vi "Read Data Source.vi"(8 "error in (no error)":errorcluster, 11 "Data Source Name":string) -> (0 "error out":errorcluster, 3 "Connection Information":T1)   [LabVIEW 2020]
uses:
  ctl/Connection Information.ctl
  <vilib>/Utility/config.llb/Read Key (String).vi
  <vilib>/Utility/config.llb/Read Key (Double).vi
  <vilib>/Utility/config.llb/Read Key (Boolean).vi
  <vilib>/Utility/config.llb/Read Key (Path).vi
  <vilib>/Utility/config.llb/NI_LVConfig.lvlib
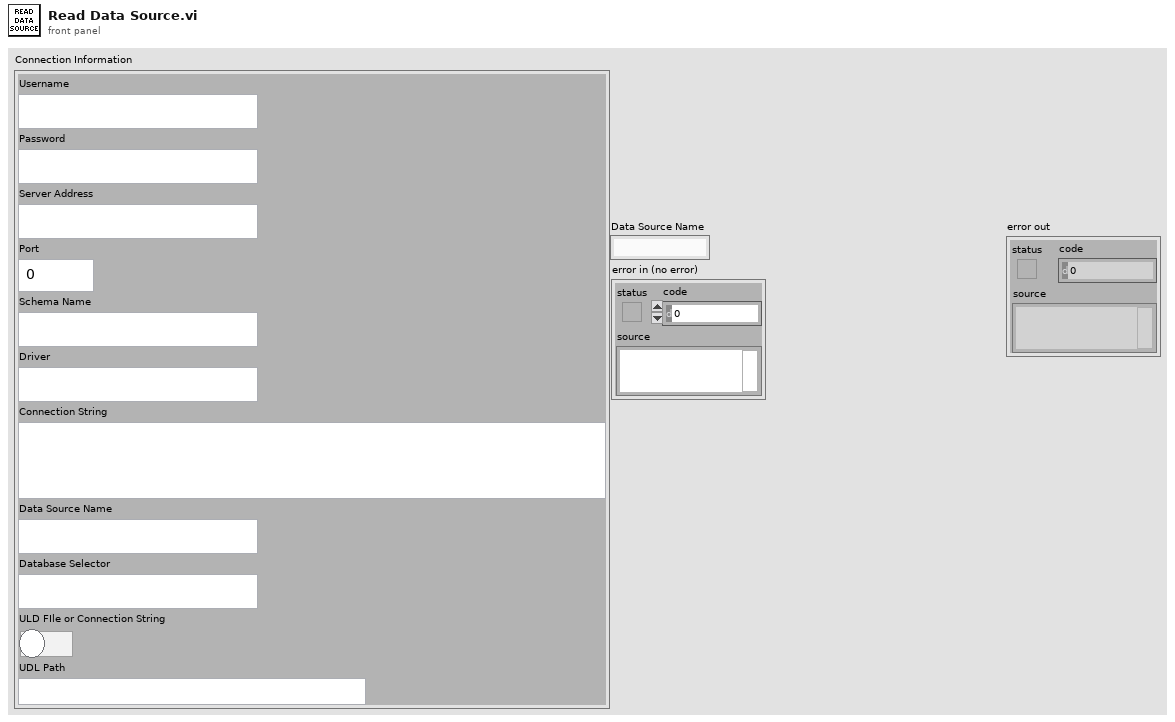
[diagram p1: front panel]
types:
  T1 = typedef "Connection Information.ctl" = cluster{"Username":string, "Password":string, "Server Address":string, "Port":u32, "Schema Name":string, "Driver":string, "Connection String":string, "Data Source Name":string, "Database Selector":string, "ULD FIle or Connection String":bool, "UDL Path":path}
  T2 = typedef "NI_LVConfig.lvlib/Config Data RefNum.ctl" = refnum<k1>
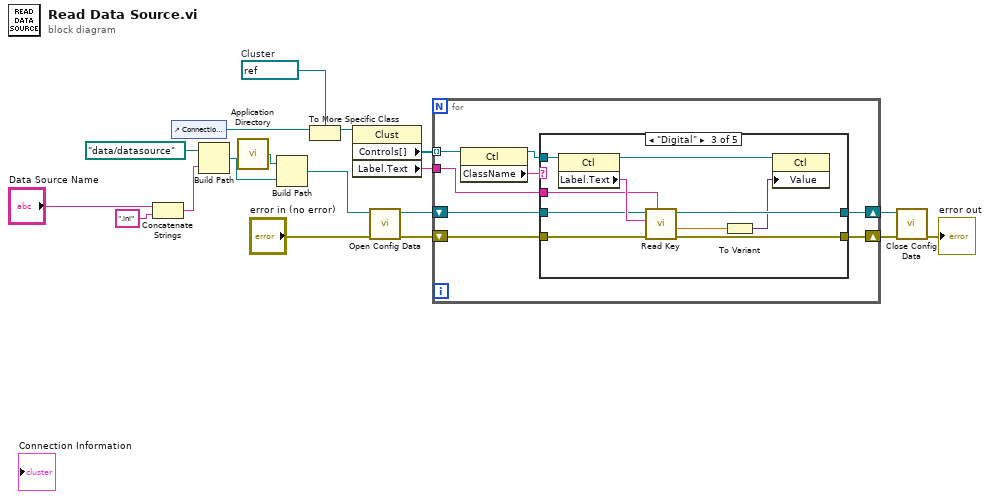
[diagram p0: block diagram]
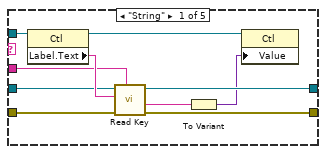
[diagram p2: hidden frame]
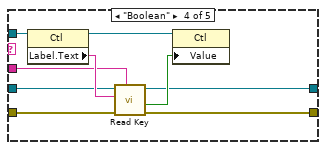
[diagram p4: hidden frame]
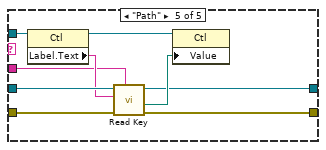
[diagram p5: hidden frame]
diagram:
  w5 = refnum<vi> refnum  # Cluster
  n1 = Concatenate Strings("Data Source Name", ".ini" ("string")) -> (w8:string)
  n2 = control-ref of="Connection Information"() -> (w1:refnum<vi>)
  n3 = Build Path(base path=path "data/datasource", name or relative path=w8) -> (appended path=w10:path)
  n4 = call <vilib>:"Application Directory.vi"() -> ("Application Directory"=w18:path)
  n5 = Build Path(base path=w18, name or relative path=w10) -> (appended path=w17:path)
  n6 = To More Specific Class(target class=w5, reference=w1) -> (specific class reference=w4:refnum<vi>)  [unwired: 1 in, 1 out]
  n7 = property class="Clust"(reference=w4) -> ("Controls[]"=w3:refnum<vi>[], "Label.Text"=w2:string)  [unwired: 1 in, 2 out]
  n8 = call <vilib>:"Open Config Data.vi"("error in (no error)"="error in (no error)", "configuration file path"=w17) -> ("error out"=w13:errorcluster, "refnum"=w14:T2)  [unwired: 7 in, 1 out]
  n9 = for {
    tunnel: w3 -> [w20] mode=indexing
    tunnel: w2 -> [w19]
    shift-right: [w22] -> w15
    shift-left: w14 -> [w25]
    shift-right: [w21] -> w16
    shift-left: w13 -> [w24]
    n10 = property class="Ctl"(reference=w20) -> (reference out=w23:refnum<vi>, "ClassName"=w26:string)  [unwired: 1 in, 1 out]
    n11 = case shown="\"Digital\"" w26 {
      tunnel: w25 -> [w32 w38 w45 w53 w65]
      tunnel: w24 -> [w33 w37 w44 w52 w64]
      tunnel: w23 -> [w34 _ w46 w54 w66]
      tunnel: [w31 w38 w43 w51 w60] -> w22
      tunnel: [w30 w37 w42 w50 w59] -> w21
      tunnel: w19 -> [w27 _ w41 w49 w58]
      frame "String" {
        n12 = property class="Ctl"(reference=w34) -> (reference out=w35:refnum<vi>, "Label.Text"=w36:string)  [unwired: 1 in, 1 out]
        n13 = call-poly <vilib>:"Read Key.vi"("section"=w27, "error in (no error)"=w33, "key"=w36, "refnum"=w32) -> ("error out"=w30:errorcluster, "value"=w28:string, "refnum out"=w31:T2)  [unwired: 4 in, 1 out]
        n14 = To Variant(anything=w28) -> (Variant=w29:variant)
        n15 = property class="Ctl"(reference=w35, "Value"=w29) -> ()  [unwired: 1 in, 2 out]
      }
      frame "", Default {
      }
      frame "Digital" {
        n16 = property class="Ctl"(reference=w46) -> (reference out=w47:refnum<vi>, "Label.Text"=w48:string)  [unwired: 1 in, 1 out]
        n17 = call-poly <vilib>:"Read Key.vi"("section"=w41, "error in (no error)"=w44, "key"=w48, "refnum"=w45) -> ("error out"=w42:errorcluster, "value"=w39:dbl, "refnum out"=w43:T2)  [unwired: 4 in, 1 out]
        n18 = To Variant(anything=w39) -> (Variant=w40:variant)
        n19 = property class="Ctl"(reference=w47, "Value"=w40) -> ()  [unwired: 1 in, 2 out]
      }
      frame "Boolean" {
        n20 = property class="Ctl"(reference=w54) -> (reference out=w56:refnum<vi>, "Label.Text"=w57:string)  [unwired: 1 in, 1 out]
        n21 = call-poly <vilib>:"Read Key.vi"("section"=w49, "error in (no error)"=w52, "key"=w57, "refnum"=w53) -> ("error out"=w50:errorcluster, "value"=w55:bool, "refnum out"=w51:T2)  [unwired: 4 in, 1 out]
        n22 = property class="Ctl"(reference=w56, "Value"=w55) -> ()  [unwired: 1 in, 2 out]
      }
      frame "Path" {
        n23 = property class="Ctl"(reference=w66) -> (reference out=w62:refnum<vi>, "Label.Text"=w63:string)  [unwired: 1 in, 1 out]
        n24 = call-poly <vilib>:"Read Key.vi"("section"=w58, "error in (no error)"=w64, "key"=w63, "refnum"=w65) -> ("error out"=w59:errorcluster, "value"=w61:path, "refnum out"=w60:T2)  [unwired: 4 in, 1 out]
        n25 = property class="Ctl"(reference=w62, "Value"=w61) -> ()  [unwired: 1 in, 2 out]
      }
    }
  }
  n26 = call <vilib>:"Close Config Data.vi"("error in (no error)"=w16, "refnum"=w15) -> ("error out"=→"error out":errorcluster)  [unwired: 8 in, 1 out]
